vi "CLD 7 Time Stamp to Initialization String exercise.vi"(8 "Fehler (Eingang)":T1) -> (0 "Fehler (Ausgang)":T1, 3 "Code-String (Ausgang)":string)   [LabVIEW 2009]
doc: "CLD-Übung 7"
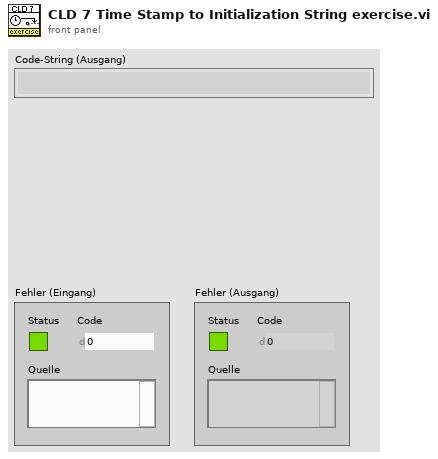
[diagram p1: front panel]
types:
  T1 = cluster{"Status":bool, "Code":i32, "Quelle":string}
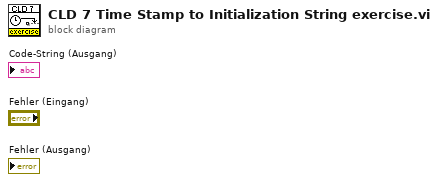
[diagram p0: block diagram]
diagram:
